vi "databasefilei_o.vi"   [LabVIEW 2019]
uses:
  <vilib>/Utility/file.llb/Write Delimited Spreadsheet (string).vi
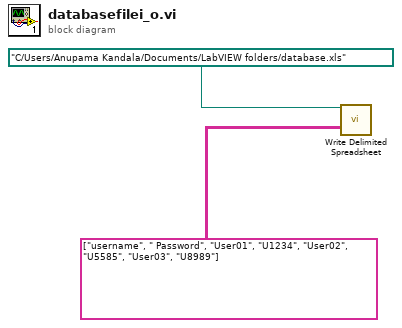
[diagram p0: block diagram]
diagram:
  n1 = call-poly <vilib>:"Write Delimited Spreadsheet.vi"("file path (dialog if empty)"=path "C:/Users/Anupama Kandala/Documents/LabVIEW folders/database.xls", "2D data"=string[][] [["username", " Password"], ["User01", "U1234"], ["User02", "U5585"], ["User03", "U8989"]]) -> ()  [unwired: 12 in, 2 out]
